vi "Set Gum Machine.vi"(0 "reference in":refnum<class "Gum Machine.lvclass">, 5 "error in (no error)":errorcluster, 6 "Number Of Gums":u32) -> (14 "reference out":refnum<class "Gum Machine.lvclass">, 19 "error out":errorcluster)   [LabVIEW 2013, in "Gum Machine.lvclass"]
uses:
  Gum Machine.lvclass
  No Coin State_class/No Coin State.lvclass
  Has Coin State_class/Has Coin State.lvclass
  Sold Out State_class/Sold Out State.lvclass
  Sold State_class/Sold State.lvclass
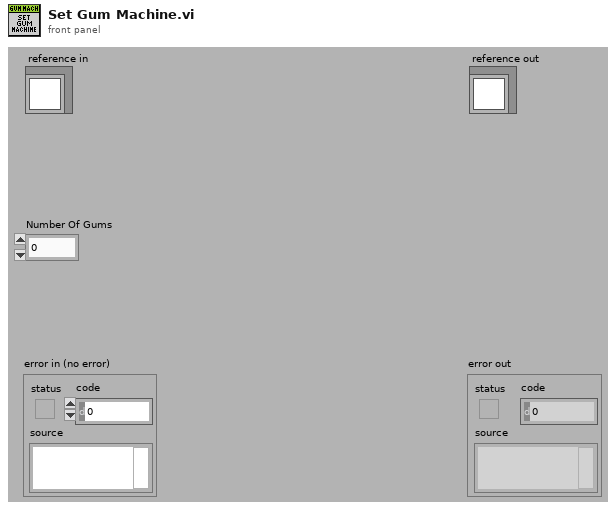
[diagram p1: front panel]
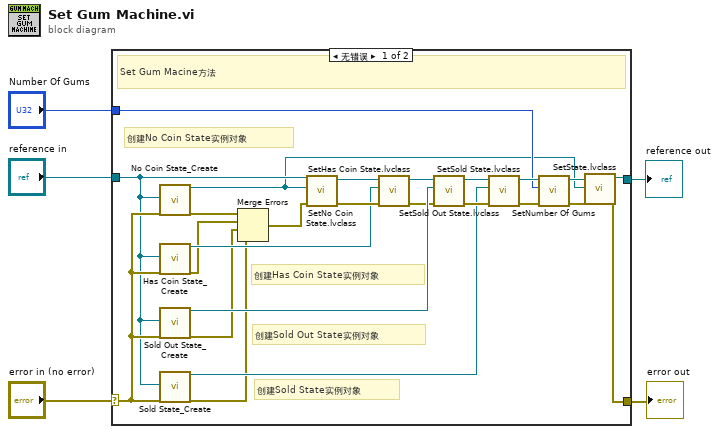
[diagram p0: block diagram]
diagram:
  n1 = case shown="无错误" "error in (no error)" {
    selector: "error in (no error)" -> [w19 w31]
    tunnel: [w7 w31] -> w4
    tunnel: [w9 w30] -> w2
    tunnel: "reference in" -> [w14 w30]
    tunnel: "Number Of Gums" -> [w11 _]
    frame No Error {
      # "创建No Coin State实例对象"
      # "创建Has Coin State实例对象"
      # "创建Sold Out State实例对象"
      # "创建Sold State实例对象"
      # "Set Gum Macine方法"
      n2 = call "No Coin State_Create.vi"("Gum Machine.lvclass"=w14, "error in (no error)"=w19) -> ("reference out"=w6:refnum<class "No Coin State.lvclass">, "error out"=w21:errorcluster)  [unwired: 16 in]
      n3 = call "Has Coin State_Create.vi"("Gum Machine.lvclass"=w14, "error in (no error)"=w19) -> ("reference out"=w28:refnum<class "Has Coin State.lvclass">, "error out"=w17:errorcluster)  [unwired: 16 in]
      n4 = call "Sold Out State_Create.vi"("Gum Machine.lvclass"=w14, "error in (no error)"=w19) -> ("reference out"=w26:refnum<class "Sold Out State.lvclass">, "error out"=w16:errorcluster)  [unwired: 16 in]
      n5 = call "Sold State_Create.vi"("Gum Machine.lvclass"=w14, "error in (no error)"=w19) -> ("reference out"=w22:refnum<class "Sold State.lvclass">, "error out"=w15:errorcluster)  [unwired: 16 in]
      n6 = Merge Errors(w21, w17, w16, w15) -> (w18:errorcluster)
      n7 = call-dynamic "SetNo Coin State.lvclass.vi"("error in (no error)"=w18, "No Coin State.lvclass"=w6, "reference in"=w14) -> ("error out"=w29:errorcluster, "reference out"=w27:refnum<class "Gum Machine.lvclass">)  [unwired: 7 in]
      n8 = call-dynamic "SetHas Coin State.lvclass.vi"("error in (no error)"=w29, "Has Coin State.lvclass"=w28, "reference in"=w27) -> ("error out"=w20:errorcluster, "reference out"=w25:refnum<class "Gum Machine.lvclass">)  [unwired: 7 in]
      n9 = call-dynamic "SetSold Out State.lvclass.vi"("error in (no error)"=w20, "Sold Out State.lvclass"=w26, "reference in"=w25) -> ("error out"=w23:errorcluster, "reference out"=w24:refnum<class "Gum Machine.lvclass">)  [unwired: 7 in]
      n10 = call-dynamic "SetSold State.lvclass.vi"("error in (no error)"=w23, "Sold State.lvclass"=w22, "reference in"=w24) -> ("error out"=w13:errorcluster, "reference out"=w12:refnum<class "Gum Machine.lvclass">)  [unwired: 7 in]
      n11 = call-dynamic "SetNumber Of Gums.vi"("error in (no error)"=w13, "Number Of Gums"=w11, "reference in"=w12) -> ("error out"=w8:errorcluster, "reference out"=w10:refnum<class "Gum Machine.lvclass">)  [unwired: 7 in]
      n12 = call-dynamic "SetState.lvclass.vi"("error in (no error)"=w8, "State.lvclass"=w6, "reference in"=w10) -> ("error out"=w7:errorcluster, "reference out"=w9:refnum<class "Gum Machine.lvclass">)  [unwired: 7 in]
    }
    frame Error {
    }
  }
  "error out" <- w4
  "reference out" <- w2
